vi "my_global.vi"() -> ()   [LabVIEW 2017]
panel:
  in  "Wordsize":u32=16
  in  "Samples":u32=1000
  in  "ChannelNum":u32=100
  # "number of channels pro worker"
  # "number of samples pro channel"
  # "resolution of ADC"
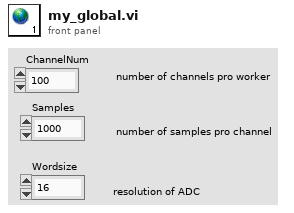
[diagram p1: front panel]
diagram:
